vi "Main.vi"() -> ()   [LabVIEW 2020]
uses:
  C:/Program Files/National Instruments/LabVIEW 2020/vi.lib/ActorFramework/Actor/Actor.lvclass
  <vilib>/ActorFramework/Actor/Actor.lvclass
panel:
  out "error out":errorcluster
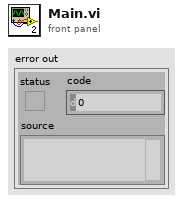
[diagram p1: front panel]
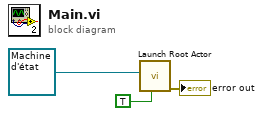
[diagram p0: block diagram]
diagram:
  n1 = call <vilib>:"Launch Root Actor.vi"("Open Actor Core front panel? (F)"=TRUE, "Actor"=refnum<class "Machine d'état.lvclass"> refnum ("Machine d'état.lvlib:Machine d'état.lvclass")) -> ("error out"=→"error out":errorcluster)  [unwired: 8 in, 1 out]
